vi "FinalizeTurn.vi"(6 "Error":errorcluster, 7 "ConcreteActor":refnum<class "ConcreteActor.lvclass">) -> (4 "Error":errorcluster, 5 "ConcreteActor":refnum<class "ConcreteActor.lvclass">)   [LabVIEW 2020, in "_Template.lvlib" / "ActorTemplate.lvlib" / "{{Name}}.lvlib" / "ConcreteActor.lvclass"]
uses:
  ConcreteActor.lvclass
  ConcreteActor.lvclass/ConcreteActor.ctl
  jettl/jettl/Actor/Actor.lvclass
panel:
  # "This front panel should not be manipulated."
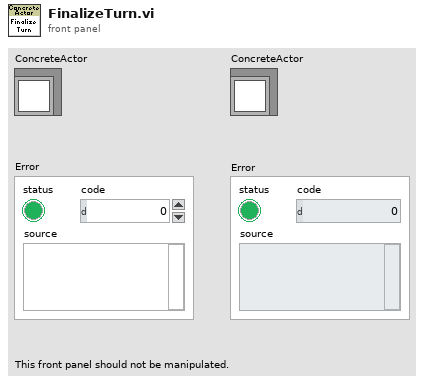
[diagram p1: front panel]
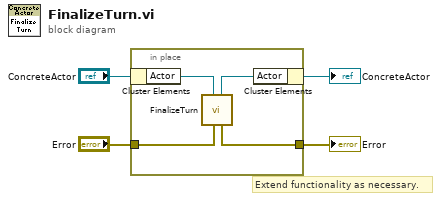
[diagram p0: block diagram]
diagram:
  # "Extend functionality as necessary."
  n1 = in-place {
    in-place-border: "Error" -> [w6]
    in-place-border: [w5] -> w1
    n2 = in-place-cluster #1("ConcreteActor") -> ("Actor"=w8:refnum<class "Actor.lvclass">)
    n3 = call-dynamic "FinalizeTurn.vi"("Error"=w6, "Actor"=w8) -> ("Error"=w5:errorcluster, "Actor"=w7:refnum<class "Actor.lvclass">)  [unwired: 8 in]
    n4 = in-place-cluster #1("Actor"=w7) -> (→"ConcreteActor":refnum<class "ConcreteActor.lvclass">)
  }
  "Error" <- w1
